vi "PNAmeas.vi"(4 "Run":refnum<vi>, 5 "Error In (no error)":errorcluster, 6 "Meas":T2, 7 "PNA Config":T1={"Sweep Type"=0, "Sweep Gen Type"=0, "Sweep Points"=1001, "Bandwidth (Hz)"=1000.0, "Center Freq (Hz)"=6000000000.0, "Span Freq (Hz)"=4000000000.0, "Power Level (dBm)"=-70.0, "Average Count"=1, "Electrical Delay (s)"=0.0} {"Electrical Delay (s)" format="%.6p"; "Power Level (dBm)" format="%.2p"; "Span Freq (Hz)" format="%.6p"; "Center Freq (Hz)" format="%.6p"; "Bandwidth (Hz)" format="%.2p"; "Sweep Gen Type" items=["Analog", "Stepped"]; "Sweep Type" items=["Linear Frequency", "Log Frequency", "Power Sweep", "CW Time"]}, 8 "VISA session":refnum<visa-resource-name>) -> (0 "Error Out":errorcluster, 1 "PNAfreq":dbl[](array[numeric]), 2 "PNAdata":dbl[][](array[numeric]), 3 "dup VISA session":refnum<visa-resource-name>)   [LabVIEW 2017]
uses:
  <instrlib>/Agilent PNA Series/Agilent PNA Series.lvlib
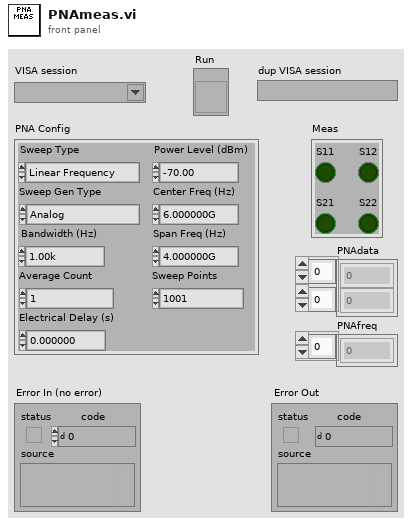
[diagram p1: front panel]
types:
  T1 = cluster{"Sweep Type":i32, "Sweep Gen Type":i32, "Sweep Points":i32, "Bandwidth (Hz)":dbl, "Center Freq (Hz)":dbl, "Span Freq (Hz)":dbl, "Power Level (dBm)":dbl, "Average Count":i32, "Electrical Delay (s)":dbl}
  T2 = cluster{"S11":bool, "S12":bool, "S21":bool, "S22":bool}
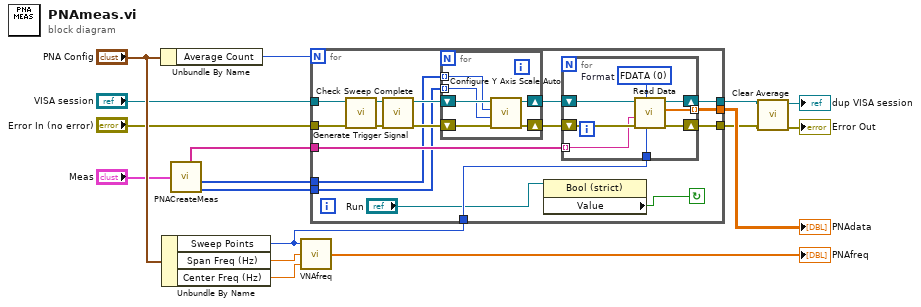
[diagram p0: block diagram]
diagram:
  n1 = Unbundle By Name("PNA Config") -> ("Average Count"=w5:i32)
  n2 = Unbundle By Name("PNA Config") -> ("Sweep Points"=w1:i32, "Span Freq (Hz)"=w17:dbl, "Center Freq (Hz)"=w16:dbl)
  n3 = call "PNACreateMeas.vi"("Meas in"="Meas") -> ("Disp traces"=w2:i32[], "Disp windows"=w3:i32[], "Meas names"=w4:string[])  [unwired: 2 out]
  n4 = call "VNAfreq.vi"("Center Freq (Hz)"=w16, "Span Freq (Hz)"=w17, "Sweep Points"=w1) -> ("VNA Freq"=→"PNAfreq":dbl[])
  n5 = for {
    N: w5 -> [_]
    tunnel: [w28] -> w9
    tunnel: "VISA session" -> [w27]
    tunnel: w1 -> [w26]
    tunnel: w4 -> [w25]
    tunnel: w3 -> [w24]
    tunnel: w2 -> [w23]
    tunnel: [w22] -> w8
    tunnel: [w21] -> w10
    tunnel: "Error In (no error)" -> [w20]
    stop <- w18 continue-if-true
    n6 = call <instrlib>:"Generate Trigger Signal.vi"("Error In (no error)"=w20, "VISA Resource Name"=w27) -> ("Error Out"=w33:errorcluster, "VISA Resource Name Out"=w34:refnum<visa-resource-name>)  [unwired: 8 in]
    n7 = call <instrlib>:"Check Sweep Complete.vi"("Error In (no error)"=w33, "VISA Resource Name"=w34) -> ("Error Out"=w29:errorcluster, "VISA Resource Name Out"=w32:refnum<visa-resource-name>)  [unwired: 7 in, 1 out]
    n8 = for {
      shift-right: [w39] -> w31
      shift-left: w32 -> [w40]
      shift-right: [w38] -> w30
      shift-left: w29 -> [w37]
      tunnel: w24 -> [w36] mode=indexing
      tunnel: w23 -> [w35] mode=indexing
      n9 = call <instrlib>:"Configure Y Axis Scale Auto.vi"("Error In (no error)"=w37, "Display Trace (1)"=w35, "Display Window (1)"=w36, "VISA Resource Name"=w40) -> ("Error Out"=w38:errorcluster, "VISA Resource Name Out"=w39:refnum<visa-resource-name>)  [unwired: 6 in]
    }
    n10 = property class="Bool (strict)"(reference="Run") -> ("Value"=w18:bool)  [unwired: 1 in, 2 out]
    n11 = for {
      tunnel: w26 -> [w45]
      shift-right: [w47] -> w21
      shift-left: w31 -> [w44]
      shift-right: [w46] -> w22
      shift-left: w30 -> [w43]
      tunnel: w25 -> [w42] mode=indexing
      tunnel: [w41] -> w28 mode=indexing
      w48 = u16 0 items=["FDATA", "SDATA", "FMEM", "SMEM", "SDIV"]  # Format
      n12 = call <instrlib>:"Read Data.vi"("Sample Count (401)"=w45, "Format  (0: FDATA)"=w48, "Error In (no error)"=w43, "Measurement Name (MY_MEAS)"=w42, "VISA Resource Name"=w44) -> ("Error Out"=w46:errorcluster, "Data"=w41:dbl[], "VISA Resource Name Out"=w47:refnum<visa-resource-name>)  [unwired: 4 in]
    }
  }
  "PNAdata" <- w9
  n13 = call <instrlib>:"Clear Average.vi"("Error In (no error)"=w8, "VISA Resource Name"=w10) -> ("Error Out"=→"Error Out":errorcluster, "VISA Resource Name Out"=→"dup VISA session":refnum<visa-resource-name>)  [unwired: 8 in]
